vi "DataPacker_ResizeQueue.vi"(8 "error in (no error)":errorcluster, 10 "max queue size (-1, unlimited)":i32, 11 "DataPacker in":refnum<class "DataPacker.lvclass">) -> (0 "error out":errorcluster, 2 "max queue size":i32, 3 "DataPacker out":refnum<class "DataPacker.lvclass">)   [LabVIEW 2018, in "feGEM DataPacker.lvlib" / "DataPacker.lvclass"]
uses:
  DataPacker.lvclass
  DataStructures/GEM_BANK_CLUSTER_typedef.ctl
  DataStructures/GEM_DATA_cluster_typedef.ctl
  DataPacker.lvclass/DataPacker.ctl
  feGEM DataPacker.lvlib
  <vilib>/Utility/SystemLogging/NI_SystemLogging.lvlib
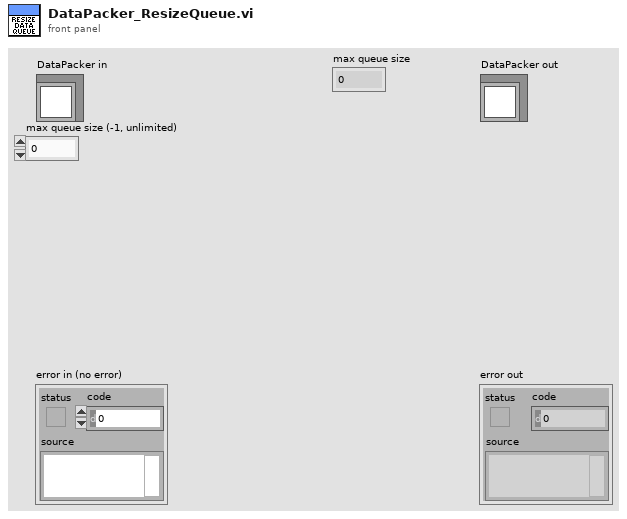
[diagram p1: front panel]
types:
  T1 = typedef "feGEM DataPacker.lvlib/GEM_BANK_CLUSTER_typedef.ctl" = cluster{"Category":string, "Variable Name":string, "Equipment description":string, "History Settings":u16, "Period to update history plots":u16, "GEM_DATA Cluster":T2}
  T2 = typedef "feGEM DataPacker.lvlib/GEM_DATA_cluster_typedef.ctl" = cluster{"DataType":string, "Formatted Data":u8[], "data byte order (Little Endian prefered)":enum16{"big-endian, network order", "native, host order", "little-endian"}}
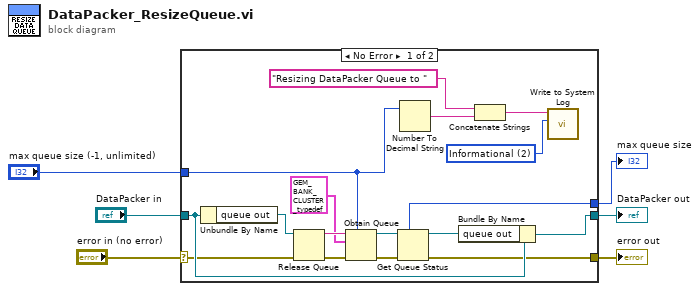
[diagram p0: block diagram]
diagram:
  n1 = case shown="No Error" "error in (no error)" {
    selector: "error in (no error)" -> [w12 w25]
    tunnel: [w15 w25] -> w5
    tunnel: [w22 w24] -> w3
    tunnel: "DataPacker in" -> [w23 w24]
    tunnel: "max queue size (-1, unlimited)" -> [w10 _]
    tunnel: [w21 _] -> w1
    frame No Error {
      w11 = 2 items=["Error", "Warning", "Informational"] ("severity")
      n2 = Unbundle By Name(w23) -> ("queue out"=w20:refnum<queue>)
      n3 = Release Queue(queue=w20, error in (no error)=w12) -> (queue name=w19:string, error out=w13:errorcluster)  [unwired: 1 in, 1 out]
      n4 = Obtain Queue(max queue size (-1, unlimited)=w10, name (unnamed)=w19, element data type=T1 {"Category"="", "Variable Name"="", "Equipment description"="", "History Settings"=0, "Period to update history plots"=0, "GEM_DATA Cluster"={"DataType"="", "Formatted Data"=[], "data byte order (Little Endian prefered)"=enum."big-endian, network order"}} ("output cluster"), error in (no error)=w13) -> (queue out=w17:refnum<queue>, error out=w14:errorcluster)  [unwired: 1 in, 1 out]
      n5 = Get Queue Status(queue=w17, error in (no error)=w14) -> (queue out=w16:refnum<queue>, max queue size=w21:i32, error out=w15:errorcluster)  [unwired: 1 in, 5 out]
      n6 = Number To Decimal String(number=w10) -> (decimal integer string=w8:string)  [unwired: 1 in]
      n7 = Bundle By Name(cluster=w23, "queue out"=w16) -> (w22:refnum<class "DataPacker.lvclass">)
      n8 = Concatenate Strings("Resizing DataPacker Queue to " ("message"), w8) -> (w7:string)
      n9 = call <vilib>:"Write to System Log.vi"("severity"=w11, "message"=w7) -> ()  [unwired: 9 in, 1 out]
    }
    frame Error {
    }
  }
  "error out" <- w5
  "DataPacker out" <- w3
  "max queue size" <- w1
